vi "sv_Get Function Type String.vi"(4 "function type":T1 items=["Signal"=0, "Speed"=3, "Ratio"=6, "Count"=7, "-"=9, "Level"=10, "-"=19, "Octave Spectrum"=20, "-"=29, "FFT Auto Spectrum"=30, "FFT Cross Spectrum"=40, "Frequency Response"=50, "-"=59, "Event"=90]) -> (1 "function type string":string)   [LabVIEW 2017]
uses:
  <vilib>/addons/_NISVFA/_Shared subVIs/Controls/NI Function Type.ctl
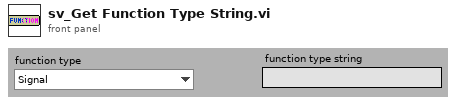
[diagram p1: front panel]
types:
  T1 = typedef "NI Function Type.ctl" = u16
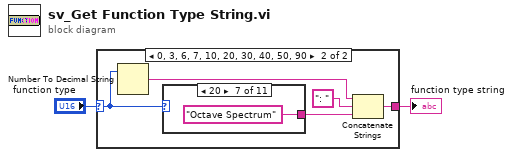
[diagram p0: block diagram]
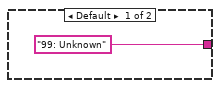
[diagram p2: hidden frame]
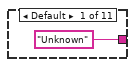
[diagram p3: hidden frame]
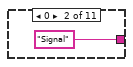
[diagram p4: hidden frame]
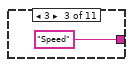
[diagram p5: hidden frame]
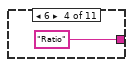
[diagram p6: hidden frame]
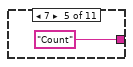
[diagram p7: hidden frame]
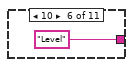
[diagram p8: hidden frame]
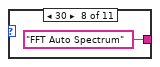
[diagram p9: hidden frame]
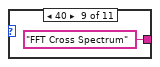
[diagram p10: hidden frame]
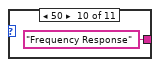
[diagram p11: hidden frame]
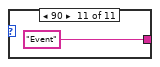
[diagram p12: hidden frame]
diagram:
  n1 = case shown="0, 3, 6, 7, 10, 20, 30, 40, 50, 90" "function type" {
    selector: "function type" -> [_ w5]
    tunnel: ["99: Unknown" ("String") w4] -> w1
    frame Default {
    }
    frame 0, 3, 6, 7, 10, 20, 30, 40, 50, 90 {
      n2 = Number To Decimal String(number=w5) -> (decimal integer string=w8:string)  [unwired: 1 in]
      n3 = case shown="20" w5 {
        tunnel: ["Unknown" ("String") "Signal" ("String") "Speed" ("String") "Ratio" ("String") "Count" ("String") "Level" ("String") "Octave Spectrum" ("String") "FFT Auto Spectrum" ("String") "FFT Cross Spectrum" ("String") "Frequency Response" ("String") "Event" ("String")] -> w6
        frame Default {
        }
        frame 0 {
        }
        frame 3 {
        }
        frame 6 {
        }
        frame 7 {
        }
        frame 10 {
        }
        frame 20 {
        }
        frame 30 {
        }
        frame 40 {
        }
        frame 50 {
        }
        frame 90 {
        }
      }
      n4 = Concatenate Strings(w8, ": " ("string"), w6) -> (w4:string)
    }
  }
  "function type string" <- w1
